vi "TDMS RT Driver VI.vi"(6 "Device Clock":string, 9 "Device Inputs FIFO":refnum<k33>, 10 "Device Outputs FIFO":refnum<k33>, 11 "Device Reference":T1 format="%.0x") -> ()   [LabVIEW 2011, in "TDMS Custom Device.lvlib"]
uses:
  TDMS Custom Device.lvlib
  <vilib>/NI Veristand/Custom Device API/Custom Device Item Ref.ctl
  <vilib>/NI Veristand/Custom Device API/Custom Device Channel Type.ctl
  <vilib>/NI Veristand/Custom Device API/Get Item Property (Path).vi
  <vilib>/NI Veristand/Custom Device API/Get Item Property (Double).vi
  <vilib>/NI Veristand/Custom Device API/Custom Device API.lvlib
  <vilib>/NI Veristand/Custom Device Tools/Custom Device Utility Library/Custom Device Utility Library.lvlib
panel:
  out "dt":dbl
  out "Channel Length":dbl
  out "# elements":u32
  in  "Status Notifier":refnum<notifier>
  # "Custom Device Template\nv1.0"
  # "Use this template as a starting point for creating a custom device code module. The input controls shown here are specially named controls that the system will use to provide the device loop with data. The controls are not required for the device loop to run. For instance, if the device doesn't produce any output data, then you don't need the Device Outputs FIFO control. If you do use these controls, however, they need to have these exact names to be functional."
  # "The optional status notifier element is used to notify the RT engine of the last state of the custom device, and to indicate the device has completed execution. If this control is not used, a default No Error value is returned to the system when the device finishes execution."
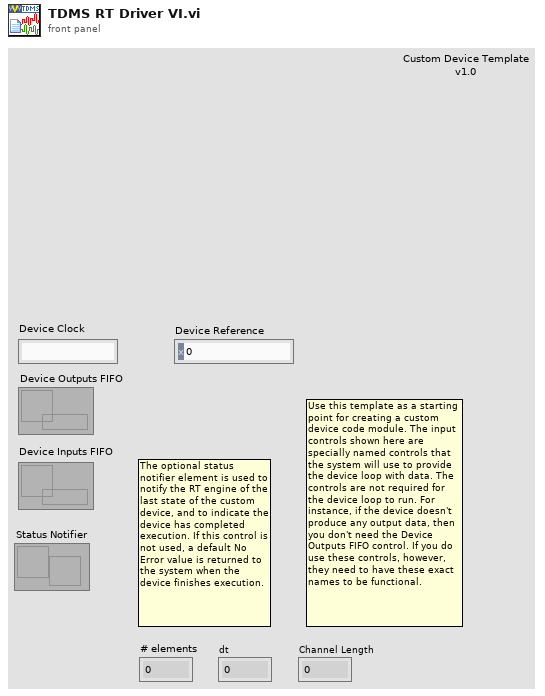
[diagram p1: front panel]
types:
  T1 = typedef "Custom Device API.lvlib/Custom Device Item Ref.ctl" = u64
  T2 = enum16{"Play and Repeat Last", "Stop (and Reset)", "Loop", "Pause"}
  T3 = typedef "Custom Device API.lvlib/Custom Device Channel Type.ctl" = enum16{"Input", "Output"}
  T4 = typedef "Custom Device API.lvlib/Custom Device Channel.ctl" = cluster{"Type":T3, "Units":string, "Default Value":dbl, "Faultable":bool, "Scalable":bool}
  T5 = enum32{"invalid OS target", "Mac OS", "Windows 3.1", "Windows 95/NT", "Solaris 1", "Solaris 2", "HP-UX", "PowerMAX", "Linux", "Irix", "Rhapsody", "BeOS", "AIX", "OSF1", "VxWorks", "PharLap", "Carbon", "RTX", "Windows x64", "Linux x64"}
  T6 = typedef "Custom Device API.lvlib/Custom Device Item Info.ctl" = cluster{"Name":string, "Is Channel":bool, "GUID":string}
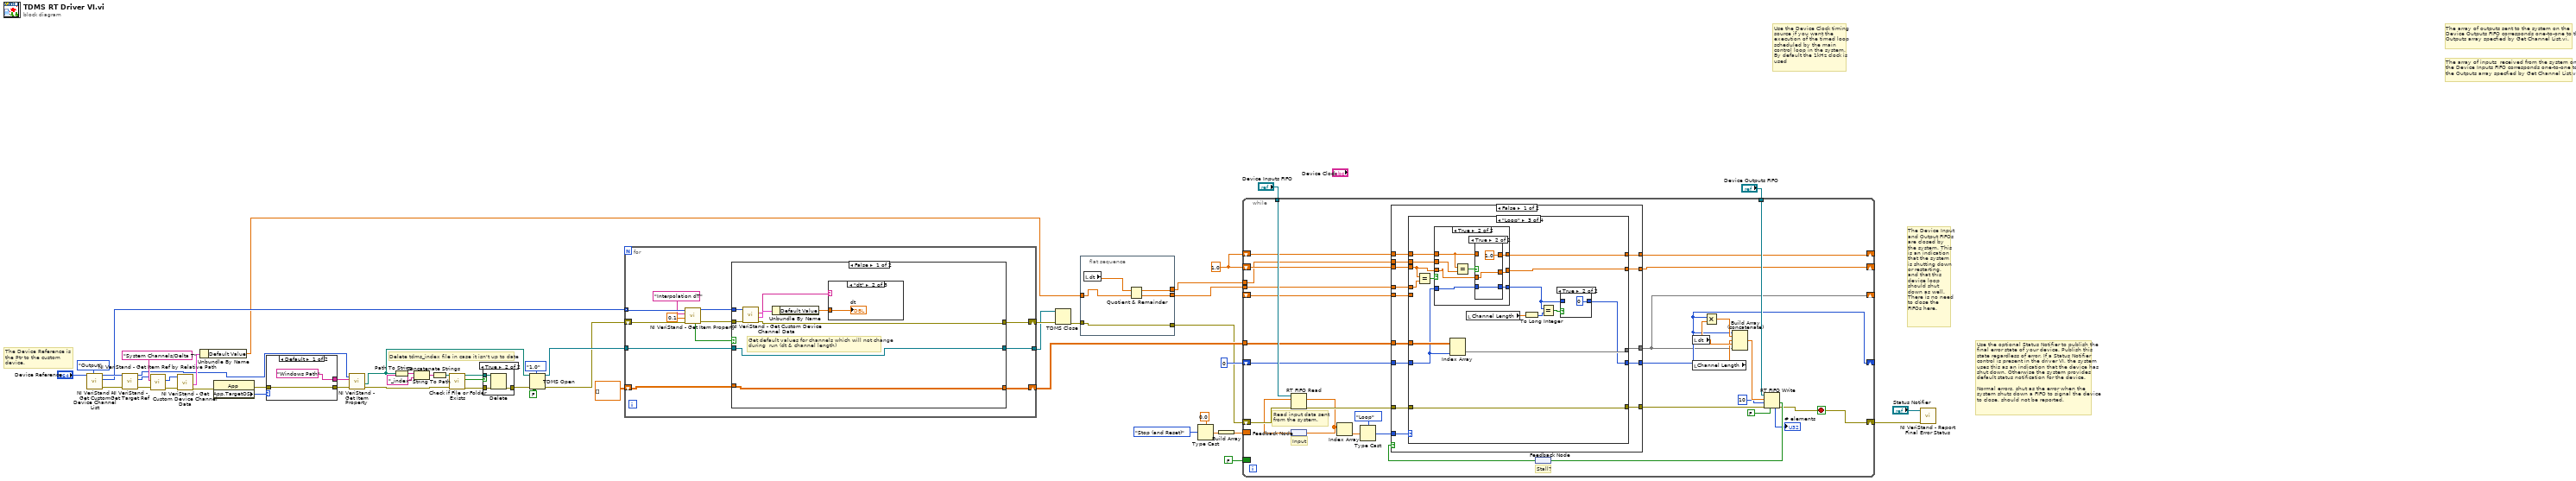
[diagram p0: block diagram]
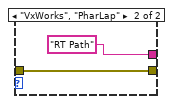
[diagram p2: hidden frame]
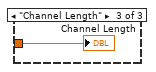
[diagram p5: hidden frame]
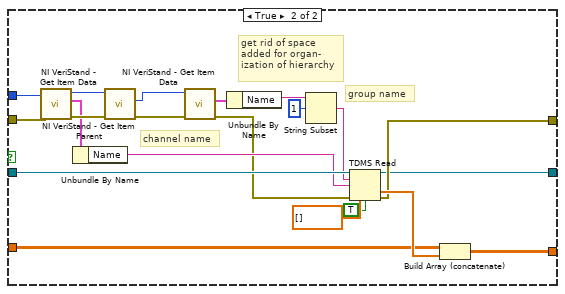
[diagram p6: hidden frame]
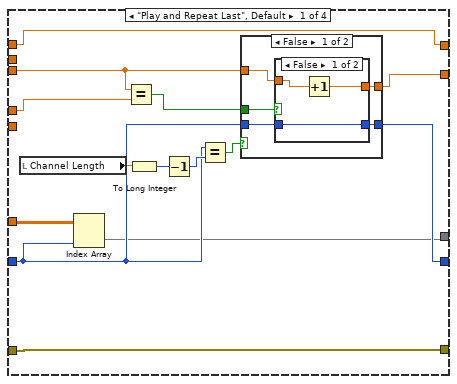
[diagram p7: hidden frame]
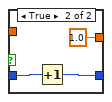
[diagram p8: hidden frame]
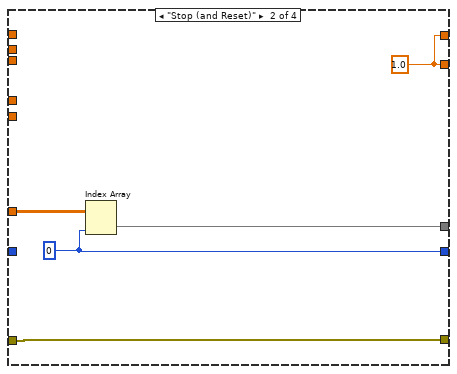
[diagram p10: hidden frame]
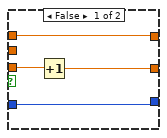
[diagram p11: hidden frame]
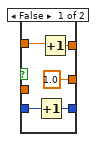
[diagram p12: hidden frame]
diagram:
  w7 = 1.0 ("Default Value")
  # "Delete tdms_index file in case it isn't up to date"
  # "The array of inputs  received from the system on the Device Inputs FIFO corresponds one-to-one to the Outputs array specfied by Get Channel List.vi."
  # "Use the optional Status Notifier to publish the final error state of your device. Publish this state regardless of error. If a Status Notifier control is present in the driver VI, the system uses this as an indication that the device has shut down. Otherwise the system provides default status notification for the device.\n\nNormal errors, shut as the error when the system shuts down a FIFO to signal the device to close, should not be reported."
  # "The Device Input and Output FIFOs are closed by the system. This is an indication that the system is shutting down or restarting, and that this device loop should shut down as well. There is no need to close the FIFOs here."
  # "The array of outputs sent to the system on the Device Outputs FIFO corresponds one-to-one to the Outputs array specfied by Get Channel List.vi."
  # "The Device Reference is\nthe Ptr to the custom device."
  # "Use the Device Clock timing source if you want the execution of the timed loop scheduled by the main control loop in the system. \nBy default the 1kHz clock is used"
  n1 = call <vilib>:"NI VeriStand - Get Custom Device Channel List.vi"("Channel Type"=Custom_Device_Channel_Type."Output", "Device Ref in"="Device Reference") -> ("error out"=w44:errorcluster, "Specified Channel Ref List"=w30:T1[], "Device Ref out"=w45:T1)  [unwired: 1 in, 6 out]
  n2 = call <vilib>:"NI VeriStand - Get Target Ref.vi"("error in"=w44, "Item Ref in"=w45) -> ("error out"=w19:errorcluster, "Target Ref"=w13:T1, "Item Ref out"=w2:T1)  [unwired: 7 out]
  n3 = call <vilib>:"NI VeriStand - Get Item Ref by Relative Path.vi"("error in"=w19, "Relative Item Path"="System Channels/Delta T", "Section Ref in"=w13) -> ("error out"=w16:errorcluster, "Item Ref"=w17:T1)  [unwired: 5 in, 2 out]
  n4 = call <vilib>:"NI VeriStand - Get Custom Device Channel Data.vi"("error in (no error)"=w16, "Channel Ref in"=w17) -> ("error out"=w15:errorcluster, "Channel"=w14:T4)  [unwired: 4 in, 4 out]
  n5 = Unbundle By Name(w14) -> ("Default Value"=w10:dbl)
  n6 = property class="App"(error in=w15) -> (error out=w6:errorcluster, "App.TargetOS"=w31:T5)  [unwired: 1 in, 1 out]
  n7 = case shown="Default" w31 {
    tunnel: [w53 w55] -> w5
    tunnel: w6 -> [w53 w55]
    tunnel: ["Windows Path" ("name or relative path") "RT Path" ("name or relative path")] -> w1
    frame Default {
    }
    frame "VxWorks", "PharLap" {
    }
  }
  n8 = call-poly <vilib>:"NI VeriStand - Get Item Property.vi"("error in (no error)"=w5, "Property Name"=w1, "Item Ref in"=w2) -> ("error out"=w4:errorcluster, "Value"=w3:path)  [unwired: 5 in, 2 out]
  n9 = Path To String(path=w3) -> (string=w33:string)
  n10 = Concatenate Strings(w33, "_index" ("name or relative path")) -> (w34:string)
  n11 = String To Path(string=w34) -> (path=w32:path)
  n12 = call <vilib>:"Check if File or Folder Exists.vi"("error in (no error)"=w4, "path"=w32) -> ("error out"=w36:errorcluster, "file or folder exists?"=w38:bool, "dup path"=w37:path)  [unwired: 7 in]
  n13 = case shown="True" w38 {
    tunnel: [w56 w59] -> w29
    tunnel: w37 -> [_ w58]
    tunnel: w36 -> [w56 w57]
    frame False {
    }
    frame True {
      n14 = Delete(path (use dialog)=w58, error in=w57) -> (error out=w59:errorcluster)  [unwired: 3 in, 2 out]
    }
  }
  n15 = TDMS Open(6:FALSE ("disable buffering (T)"), 7:enum16{"1.0", "2.0"}."1.0" ("file format version (2.0)"), 8:w29, 11:w3) -> (0:w27:errorcluster, 3:w28:refnum<k34>)  [unwired: 2 in]
  n16 = for {
    tunnel: w30 -> [w68] mode=indexing
    shift-right: [w71] -> w22
    shift-left: w27 -> [w67]
    tunnel: w28 -> [w65]
    shift-right: [w64] -> w20
    shift-left: dbl[][] [] -> [w63]
    tunnel: [w62] -> w21
    n17 = call-poly <vilib>:"NI VeriStand - Get Item Property.vi"("error in (no error)"=w67, "Default Value"=0.1, "Property Name"="Interpolation dT", "Item Ref in"=w68) -> ("error out"=w69:errorcluster, "Item Ref out"=w70:T1, "Found?"=w66:bool)  [unwired: 5 out]
    n18 = case shown="False" w66 {
      tunnel: [w74 w84] -> w71
      tunnel: w70 -> [w79 w101]
      tunnel: w69 -> [w78 w102]
      tunnel: w65 -> [w72 w92]
      tunnel: [w73 w86] -> w64
      tunnel: w63 -> [w73 w85]
      tunnel: [w72 w83] -> w62
      frame False {
        # "Get default values for channels which will not change during  run (dt & channel length)"
        n19 = call <vilib>:"NI VeriStand - Get Custom Device Channel Data.vi"("error in (no error)"=w78, "Channel Ref in"=w79) -> ("error out"=w74:errorcluster, "Channel"=w77:T4, "Channel Name"=w76:string)  [unwired: 4 in, 3 out]
        n20 = Unbundle By Name(w77) -> ("Default Value"=w75:dbl)
        n21 = case shown="\"dt\"" w76 {
          tunnel: w75 -> [_ w80 w81]
          frame "", Default {
          }
          frame "dt" {
            "dt" <- w80
          }
          frame "Channel Length" {
            "Channel Length" <- w81
          }
        }
      }
      frame True {
        # "channel name"
        # "group name"
        # "get rid of space\nadded for organ-\nization of hierarchy"
        n22 = call <vilib>:"NI VeriStand - Get Item Data.vi"("error in (no error)"=w102, "Item Ref in"=w101) -> ("error out"=w100:errorcluster, "Item Info"=w95:T6, "Item Ref out"=w99:T1)  [unwired: 6 in, 1 out]
        n23 = Unbundle By Name(w95) -> ("Name"=w90:string)
        n24 = call <vilib>:"NI VeriStand - Get Item Parent.vi"("error in (no error)"=w100, "Item Ref in"=w99) -> ("error out"=w98:errorcluster, "Parent Ref"=w97:T1)  [unwired: 6 in, 2 out]
        n25 = call <vilib>:"NI VeriStand - Get Item Data.vi"("error in (no error)"=w98, "Item Ref in"=w97) -> ("error out"=w89:errorcluster, "Item Info"=w96:T6)  [unwired: 6 in, 2 out]
        n26 = Unbundle By Name(w96) -> ("Name"=w94:string)
        n27 = String Subset(string=w94, offset (0)=1) -> (substring=w91:string)  [unwired: 1 in]
        n28 = TDMS Read(0:w92, 5:w91, 7:w90, 11:w89, 12:dbl[] [], 13:TRUE ("return channels in file order? (F)")) -> (4:w83:refnum<k34>, 10:w87:dbl[], 15:w84:errorcluster)  [unwired: 2 in, 3 out]
        n29 = Build Array (concatenate)(w85, w87) -> (w86:dbl[][])
      }
    }
  }
  n30 = TDMS Close(8:w22, 11:w21) -> (0:w12:errorcluster)  [unwired: 1 out]
  n31 = flat-sequence {
    tunnel: w12 -> [w107]
    tunnel: [w107] -> w11
    tunnel: w10 -> [w105]
    tunnel: [w104] -> w9
    tunnel: [w103] -> w8
    frame #0 {
      n32 = local read "dt"() -> (w106:dbl)
      n33 = Quotient & Remainder(x=w106, y=w105) -> (x-y*floor(x/y)=w103:dbl, floor(x/y)=w104:dbl)
    }
  }
  n34 = Type Cast(type=0.0 ("element"), x=T2."Stop (and Reset)") -> (*(type *) &x=w41:dbl)
  n35 = Build Array(w41) -> (w43:dbl[])
  n36 = while {
    shift-right: [w118] -> w23
    shift-left: w11 -> [w138]
    tunnel: "Device Inputs FIFO" -> [w137]
    border: w43 -> [_]
    border: FALSE ("timed out?") -> [_]
    tunnel: w20 -> [w130]
    shift-right: [w116] -> _
    shift-left: 0 -> [w129]
    tunnel: "Device Outputs FIFO" -> [w128]
    shift-right: [w114] -> _
    shift-left: _ -> [w117]
    tunnel: w9 -> [w113]
    shift-right: [w111] -> _
    shift-left: w7 -> [w112]
    tunnel: w8 -> [w108]
    shift-right: [w109] -> _
    shift-left: w7 -> [w110]
    stop <- w118 stop-if-true
    # "Read input data sent\nfrom the system."
    # "Input"
    # "Stall?"
    n37 = feedback #1() -> (w135:dbl[])
    n38 = RT FIFO Read(0:w137, 1:w135, 3:w138) -> (9:w132:dbl[], 11:w136:errorcluster)  [unwired: 4 out]
    n39 = feedback-in #1(w132) -> ()
    n40 = Index Array(array=w132) -> (element=w134:dbl)  [unwired: 1 in]
    n41 = Type Cast(type=T2."Loop", x=w134) -> (*(type *) &x=w131:T2)
    n42 = feedback #2() -> (w120:bool)
    n43 = case shown="False" w120 {
      tunnel: w136 -> [w152 w231]
      tunnel: w131 -> [w151 _]
      tunnel: w130 -> [w150 _]
      tunnel: w129 -> [w149 w232]
      tunnel: [w148 w231] -> w127
      tunnel: [w147 w230] -> w114
      tunnel: [w146 w232] -> w116
      tunnel: w117 -> [w145 w230]
      tunnel: w113 -> [w144 _]
      tunnel: w112 -> [w143 w229]
      tunnel: [w142 w229] -> w111
      tunnel: w110 -> [w141 w228]
      tunnel: [w140 w228] -> w109
      tunnel: w108 -> [w139 _]
      frame False {
        n44 = case shown="\"Loop\"" w151 {
          tunnel: w150 -> [w161 w184 w200 _]
          tunnel: w149 -> [w160 _ w196 w227]
          tunnel: [w162 w183 w193 w227] -> w146
          tunnel: [w159 w182 w199 w225] -> w147
          tunnel: w152 -> [w158 w181 w198 w226]
          tunnel: [w158 w181 w198 w226] -> w148
          tunnel: w145 -> [_ _ _ w225]
          tunnel: w144 -> [w157 _ w189 _]
          tunnel: w143 -> [w155 _ w191 w224]
          tunnel: [w154 w180 w190 w224] -> w142
          tunnel: w141 -> [w153 _ w187 w223]
          tunnel: [w153 w180 w186 w223] -> w140
          tunnel: w139 -> [_ _ w185 _]
          frame "Play and Repeat Last", Default {
            n45 = local read "Channel Length"() -> (w166:dbl)
            n46 = Index Array(array=w161, index (col)=w160) -> (element=w159:dbl[])  [unwired: 1 in]
            n47 = Equal?(x=w155, y=w157) -> (x = y?=w156:bool)
            n48 = To Long Integer(number=w166) -> (32bit integer=w165:i32)
            n49 = Decrement(x=w165) -> (x-1=w164:i32)
            n50 = Equal?(x=w160, y=w164) -> (x = y?=w163:bool)
            n51 = case shown="False" w163 {
              tunnel: w160 -> [w171 w179]
              tunnel: [w170 w179] -> w162
              tunnel: w156 -> [w169 _]
              tunnel: w155 -> [w168 w178]
              tunnel: [w167 w178] -> w154
              frame False {
                n52 = case shown="False" w169 {
                  tunnel: w171 -> [w174 w177]
                  tunnel: [w174 w176] -> w170
                  tunnel: w168 -> [w173 _]
                  tunnel: [w172 1.0] -> w167
                  frame False {
                    n53 = Increment(x=w173) -> (x+1=w172:dbl)
                  }
                  frame True {
                    n54 = Increment(x=w177) -> (x+1=w176:i32)
                  }
                }
              }
              frame True {
              }
            }
          }
          frame "Stop (and Reset)" {
            w180 = 1.0 ("Default Value")
            w183 = 0
            n55 = Index Array(array=w184, index (col)=w183) -> (element=w182:dbl[])  [unwired: 1 in]
          }
          frame "Loop" {
            n56 = Equal?(x=w191, y=w189) -> (x = y?=w188:bool)
            n57 = case shown="True" w188 {
              tunnel: w196 -> [w204 w212]
              tunnel: [w204 w211] -> w194
              tunnel: w191 -> [w203 w205]
              tunnel: [w202 w210] -> w190
              tunnel: w187 -> [w201 w207]
              tunnel: [w201 w209] -> w186
              tunnel: w185 -> [_ w206]
              frame False {
                n58 = Increment(x=w203) -> (x+1=w202:dbl)
              }
              frame True {
                n59 = Equal?(x=w207, y=w206) -> (x = y?=w208:bool)
                n60 = case shown="True" w208 {
                  tunnel: w212 -> [w217 w218]
                  tunnel: [w216 w218] -> w211
                  tunnel: [1.0 w219] -> w210
                  tunnel: w207 -> [w214 _]
                  tunnel: [w213 1.0] -> w209
                  tunnel: w205 -> [_ w219]
                  frame False {
                    n61 = Increment(x=w217) -> (x+1=w216:i32)
                    n62 = Increment(x=w214) -> (x+1=w213:dbl)
                  }
                  frame True {
                  }
                }
              }
            }
            n63 = Index Array(array=w200, index (col)=w196) -> (element=w199:dbl[])  [unwired: 1 in]
            n64 = local read "Channel Length"() -> (w197:dbl)
            n65 = To Long Integer(number=w197) -> (32bit integer=w192:i32)
            n66 = Equal?(x=w194, y=w192) -> (x = y?=w195:bool)
            n67 = case shown="True" w195 {
              tunnel: w194 -> [w221 _]
              tunnel: [w221 0] -> w193
              frame False {
              }
              frame True {
              }
            }
          }
          frame "Pause" {
          }
        }
      }
      frame True {
        # "Spin until space\nin FIFO"
      }
    }
    n68 = local read "Channel Length"() -> (w124:dbl)
    n69 = local read "dt"() -> (w125:dbl)
    n70 = Multiply(x=w116, y=w125) -> (x*y=w126:dbl)
    n71 = Build Array (concatenate)(w116, w126, w124, w125, w114) -> (w123:dbl[])
    n72 = RT FIFO Write(0:w128, 1:w123, 2:10 ("timeout in ms (0)"), 3:w127, 5:FALSE ("overwrite on timeout (T)")) -> (7:→"# elements":u32, 10:w119:bool, 11:w118:errorcluster)  [unwired: 1 out]
    n73 = feedback-in #2(w119) -> ()
  }
  n74 = call <vilib>:"NI VeriStand - Report Final Error Status.vi"("error in (no error)"=w23, "Status Notifier"="Status Notifier") -> ()  [unwired: 1 in, 9 out]
